vi "Log Event.vi"(8 "error in":errorcluster, 10 "Event Data":T1, 11 "TDMS in":refnum<class "TDMS.lvclass">) -> (0 "error out":errorcluster, 3 "TDMS out":refnum<class "TDMS.lvclass">)   [LabVIEW 2019, in "TDMS.lvlib" / "TDMS.lvclass"]
uses:
  TDMS.lvclass
  builds/Tools/Report.lvlibp/Custom Controls/Event Data.ctl
  TDMS.lvclass/TDMS.ctl
  builds/Tools/Report.lvlibp/Report.lvclass
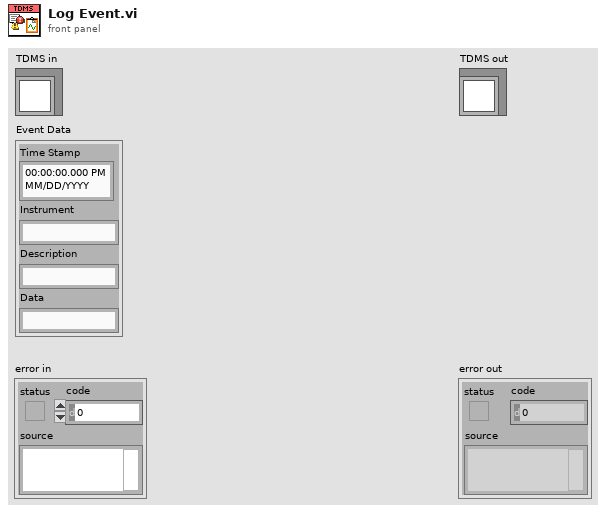
[diagram p1: front panel]
types:
  T1 = typedef "Report.lvlibp/Report.lvclass/Event Data.ctl" = cluster{"Time Stamp":timestamp, "Instrument":string, "Description":string, "Data":string}
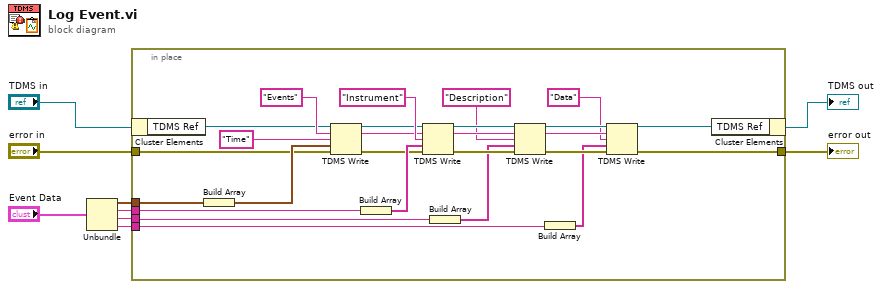
[diagram p0: block diagram]
diagram:
  n1 = Unbundle("Event Data") -> ("Time Stamp"=w4:timestamp, "Instrument"=w3:string, "Description"=w2:string, "Data"=w1:string)
  n2 = in-place {
    in-place-border: w4 -> [w35]
    in-place-border: [w20] -> w9
    in-place-border: "error in" -> [w25]
    in-place-border: w3 -> [w24]
    in-place-border: w2 -> [w15]
    in-place-border: w1 -> [w13]
    n3 = in-place-cluster #1("TDMS in") -> ("TDMS Ref"=w26:refnum<k34>)
    n4 = Build Array(w35) -> (w29:timestamp[])
    n5 = TDMS Write(0:w26, 5:"Events" ("group name"), 7:"Time" ("channel name"), 9:w29, 11:w25) -> (4:w31:refnum<k34>, 6:w30:string, 15:w32:errorcluster)  [unwired: 1 in, 1 out]
    n6 = Build Array(w24) -> (w34:string[])
    n7 = TDMS Write(0:w31, 5:w30, 7:"Instrument" ("channel name"), 9:w34, 11:w32) -> (4:w23:refnum<k34>, 6:w17:string, 15:w18:errorcluster)  [unwired: 1 in, 1 out]
    n8 = Build Array(w15) -> (w14:string[])
    n9 = TDMS Write(0:w23, 5:w17, 7:"Description" ("channel name"), 9:w14, 11:w18) -> (4:w22:refnum<k34>, 6:w16:string, 15:w19:errorcluster)  [unwired: 1 in, 1 out]
    n10 = Build Array(w13) -> (w12:string[])
    n11 = TDMS Write(0:w22, 5:w16, 7:"Data" ("channel name"), 9:w12, 11:w19) -> (4:w21:refnum<k34>, 15:w20:errorcluster)  [unwired: 1 in, 2 out]
    n12 = in-place-cluster #1("TDMS Ref"=w21) -> (→"TDMS out":refnum<class "TDMS.lvclass">)
  }
  "error out" <- w9
